vi "3.3.vi"() -> ()   [LabVIEW 2017]
panel:
  out "输出 1":dbl
  out "子字符串":string
  in  "初始扫描位置":u32
  in  "长度（剩余）":i32
  in  "偏移量(0)":i32
  in  "字符串":string
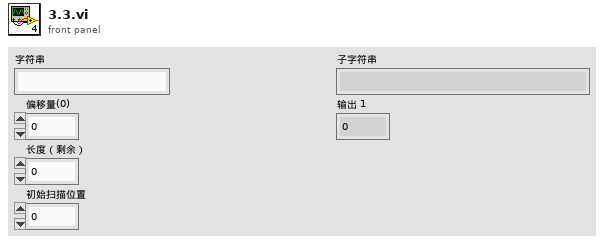
[diagram p1: front panel]
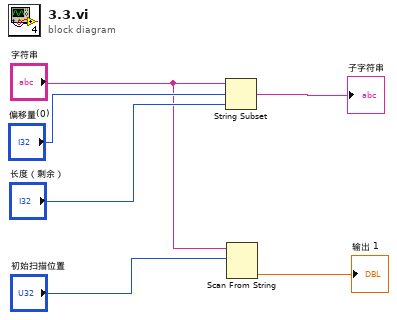
[diagram p0: block diagram]
diagram:
  n1 = String Subset(string="字符串", offset (0)="偏移量(0)", length (rest)="长度（剩余）") -> (substring=→"子字符串":string)
  n2 = Scan From String(input string="字符串", initial scan location="初始扫描位置") -> (output 1=→"输出 1":dbl)  [unwired: 3 in, 3 out]
